vi "Square_MA.vi"(1 "Input Array":dbl[](array[numeric]), 2 "L":u16=2) -> (0 "Output Array":dbl[](array[numeric]))   [LabVIEW 2023]
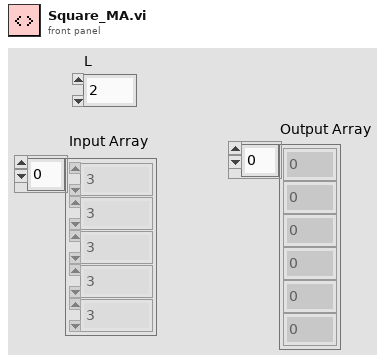
[diagram p1: front panel]
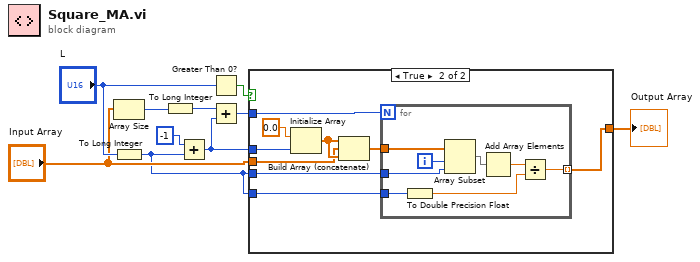
[diagram p0: block diagram]
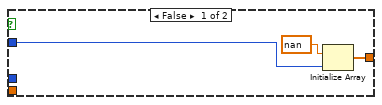
[diagram p2: hidden frame]
diagram:
  n1 = Array Size(array="Input Array") -> (size(s)=w6:i32)
  n2 = To Long Integer(number="L") -> (32bit integer=w5:i32)
  n3 = To Long Integer(number=w6) -> (32bit integer=w2:i32)
  n4 = Add(x=-1 ("value"), y=w5) -> (x+y=w3:i32)
  n5 = Greater Than 0?(x="L") -> (x > 0?=w9:bool)
  n6 = Add(x=w2, y=w3) -> (x+y=w1:i32)
  n7 = case shown="True" w9 {
    tunnel: [w12 w20] -> w8
    tunnel: "Input Array" -> [_ w19]
    tunnel: w5 -> [_ w18]
    tunnel: w5 -> [_ w17]
    tunnel: w3 -> [_ w16]
    tunnel: w1 -> [w13 w15]
    frame False {
      n8 = Initialize Array(nan, w13) -> (w12:dbl[])
    }
    frame True {
      n9 = Initialize Array(0.0 ("element"), w16) -> (w21:dbl[])
      n10 = Build Array (concatenate)(w21, w19, w21) -> (w14:dbl[])
      n11 = for {
        N: w15 -> [_]
        tunnel: w14 -> [w30]
        tunnel: [w27] -> w20 mode=indexing
        tunnel: w18 -> [w24]
        tunnel: w17 -> [w23]
        i -> [w25]
        n12 = To Double Precision Float(number=w23) -> (double precision float=w26:dbl)
        n13 = Array Subset(array=w30, index=w25, length=w24) -> (w29:dbl[])
        n14 = Add Array Elements(numeric array=w29) -> (sum=w28:dbl)
        n15 = Divide(x=w28, y=w26) -> (x/y=w27:dbl)
      }
    }
  }
  "Output Array" <- w8
